vi "Halvorsen_ECD3_Fast.vi"(0 "tolerance":dbl=1e-13, 1 "Error Analysis":u16(ring)=4 items=["Max", "Max_Norm", "Norm", "Last Value", "Last Constant"], 3 "Шаг h, с":dbl=0.01, 4 "k":i32=4, 5 "Время, с":dbl=30.0, 7 "Hmax":dbl=1.0, 8 "b":dbl[](array[numeric])=[0.1, 0.1, 0.1], 10 "last_point_Thomas":dbl[](array[numeric])=[2.3727475682665875, 0.23609824454436878, 0.4447912442126299], 13 "Hmin":dbl=0.001, 15 "Points count":i32=2, 18 "n":i32[](array[numeric])=[2, 4, 6, 8, 10, 12, 14, 16, 18, 20, 22], 19 "Ext.Type":u16(ring) items=["FNode", "MathScript", "ECD8 Arrays", "ECD8 Fnode", "ECD8 FnodeDiv", "FNode Exp"]) -> (6 "Elapsed Time":dbl=0.0023101388233044418, 12 "Number of steps":i32=215, 14 "Error Estimation":dbl=7.276980385616179e-13, 17 "Rejected steps":i32=3)   [LabVIEW 2016]
uses:
  <vilib>/Analysis/_algsub.llb/Real Vector Norm.vi
  <vilib>/Analysis/5stat.llb/RMS (DBL).vi
  <vilib>/Analysis/NI_AALBase.lvlib
  <vilib>/Analysis/NI_AALPro.lvlib
panel:
  in  "Initial Conditions":dbl[](array[numeric])=[1.0, 0.0, 1.0]
  out "Last Value Reference":dbl[](array[numeric])=[2.372747587228327, 0.2360982570449824, 0.44479123342230803] format="%#_15f"
  out "Rejected Steps":i32[](graph)=[0, 0, 0, 0, 0, 0, 0, 0, 0, 0, 0, 0, 0, 0, 0, 0, 0, 0, 0, 0, 0, 0, 0, 0, 0, 0, 0, 0, 0, 0, 0, 0, 0, 0, 0, 0, 0, 0, 0, 0, 0, 0, 0, 0, 0, 0, 0, 0, 0, 0, 0, 0, 0, 0, 0, 0, 0, 0, 0, 0, 0, 0, 0, 0, 0, 0, 0, 0, 0, 0, 0, 0, 0, 0, 0, 0, 0, 0, 0, 0, 0, 0, 0, 0, 0, 0, 0, 0, 0, 0, 0, 0, 0, 0, 0, 0, 0, 0, 0, 0, 0, 0, 0, 0, 0, 0, 0, 0, 0, 0, 0, 0, 0, 0, 1, 0, 0, 0, 0, 0, 0, 0, 0, 0, 0, 0, 0, 0, 0, 0, 0, 0, 0, 0, 0, 0, 0, 0, 0, 0, 0, 0, 0, 0, 0, 0, 0, 0, 0, 0, 0, 0, 0, 0, 0, 0, 0, 0, 0, 0, 0, 0, 0, 0, 0, 0, 0, 0, 0, 0, 0, 0, 0, 0, 0, 0, 0, 0, 0, 0, 0, 0, 0, 0, 0, 0, 1, 0, 0, 0, 0, 1, 0, 0, 0, 0, 0, 0, 0, 0, 0, 0, 0, 0, 0, 0, 0, 0, 0, 0, 0, 0, 0, 0, 0, 0]
  out "Last Value":dbl[](array[numeric])=[2.3727475682670662, 0.2360982445444861, 0.44479124421209454] format="%#_15f"
  out "Step time variation":dbl[](graph)=[0.002410370462712308, 0.0022099071838965756]
  out "Real Error":dbl[][](graph)=[[0.0, 0.0, 0.0], [4.6629367034256575e-15, 1.908195823574488e-15, 1.7763568394002505e-15], [1.748490241482159e-12, 5.903055821931957e-13, 2.1094237467877974e-14], [5.741995767749586e-11, 1.6126516788617096e-11, 1.5851764345597985e-12], [2.8038460442303403e-10, 6.303146893316125e-11, 1.404787397518703e-11], [4.9621040609793e-10, 9.647355136976898e-11, 4.231348604832874e-11], [6.795632945255647e-10, 1.172824615203183e-10, 8.282352581545638e-11], [8.33989544091196e-10, 1.2820922101752785e-10, 1.3152390287984872e-10], [9.677894041715263e-10, 1.2962053652643135e-10, 1.8526247202999002e-10], [1.087936851718041e-09, 1.1890322060281733e-10, 2.4136426191034843e-10], [1.1999332638623628e-09, 8.893674685594988e-11, 2.966178413998932e-10], [1.2968486284847813e-09, 2.879207983141896e-11, 3.4188940567503323e-10], [1.3438086199357713e-09, -4.558087240980058e-11, 3.5787728336345026e-10], [1.3577134971853866e-09, -1.2493472922869842e-10, 3.432942818903939e-10], [1.354880652115753e-09, -2.1241652881087703e-10, 2.9695623737779897e-10], [1.3423706590742768e-09, -3.1278557521829953e-10, 2.0913804021915894e-10], [1.3237086982087476e-09, -4.3100079061275665e-10, 5.410383252524298e-11], [1.3041514534961607e-09, -5.177385187238315e-10, -1.521587300601368e-10], [1.2894871836977018e-09, -5.417550852371278e-10, -3.6701575112374485e-10], [1.2790746239943473e-09, -5.146085779728082e-10, -6.057510049117809e-10], [1.2707515040233375e-09, -4.3312020636676607e-10, -8.863207945353224e-10], [1.2613066147082463e-09, -2.8478619462646293e-10, -1.2270384708301663e-09], [1.2457230802453978e-09, -5.0502935167173746e-11, -1.6514722922522651e-09], [1.2178640318438738e-09, 2.7474467145793824e-10, -2.1226838065047104e-09], [1.173521724240345e-09, 6.642104644072333e-10, -2.548607991315066e-09], [1.1083001183465058e-09, 1.1039147373992364e-09, -2.922341035827003e-09], [1.017403494785185e-09, 1.5845043055406904e-09, -3.240587354014224e-09], [8.940710394256257e-10, 2.1000174932339633e-09, -3.5038705270551418e-09], [7.26753324187257e-10, 2.650429875572513e-09, -3.716026153455232e-09], [5.006035586063717e-10, 3.2262850169217927e-09, -3.8690446402256384e-09], [1.9380763660592493e-10, 3.816509774878796e-09, -3.955048732962041e-09], [-2.0528290178845054e-10, 4.372683548581335e-09, -3.95721366786006e-09], [-6.853815293084153e-10, 4.834492361993625e-09, -3.873784404362368e-09], [-1.231378554678031e-09, 5.183864892899237e-09, -3.718152896681204e-09], [-1.838136309828542e-09, 5.43066525082736e-09, -3.4995242259583392e-09], [-2.4965642886343176e-09, 5.583902229489013e-09, -3.2218598899902418e-09], [-3.20633031236639e-09, 5.655568013906986e-09, -2.8814779451380446e-09], [-3.95173493927814e-09, 5.653833845542522e-09, -2.475329274886917e-09], [-4.717421564492952e-09, 5.591174190300308e-09, -1.997236598327845e-09], [-5.481618714497927e-09, 5.484983578440961e-09, -1.4417773641639542e-09], [-6.222447002102172e-09, 5.3586233228486435e-09, -8.048868238574869e-10], [-6.927526552402696e-09, 5.2384971915842016e-09, -8.118239414045547e-11], [-7.589623596260253e-09, 5.152425153198692e-09, 7.313869510028326e-10], [-8.214809277262702e-09, 5.1254382960053135e-09, 1.639219426863292e-09], [-8.815759233726794e-09, 5.180855744413293e-09, 2.651973751710557e-09], [-9.412382873108527e-09, 5.342479347802964e-09, 3.7888571169375496e-09], [-1.0020086094186809e-08, 5.634394728559755e-09, 5.058699126259114e-09], [-1.0670280659041964e-08, 6.0878764251981465e-09, 6.5014074124292165e-09], [-1.1386144471714488e-08, 6.732222335159577e-09, 8.133392848108656e-09], [-1.2184061315423378e-08, 7.58216733842687e-09, 9.939812195547404e-09], [-1.3073527593832068e-08, 8.631241499301723e-09, 1.1878749317517645e-08], [-1.4058679997930312e-08, 9.855596339036765e-09, 1.3899611461809513e-08], [-1.5135776632035913e-08, 1.1216054751628235e-08, 1.5948250164932176e-08], [-1.6288862259017378e-08, 1.2655923420368254e-08, 1.7962675902261083e-08], [-1.748360478615041e-08, 1.4096415590358902e-08, 1.9864868083807607e-08], [-1.8675936797052373e-08, 1.5452399360071922e-08, 2.158286260822706e-08], [-1.9839095699580866e-08, 1.6667154767446846e-08, 2.3089951728394453e-08], [-2.095904472199095e-08, 1.7701697885286194e-08, 2.437547474976043e-08], [-2.201700777249016e-08, 1.8510371013746862e-08, 2.5409759407679644e-08], [-2.300580370651062e-08, 1.904587509926614e-08, 2.615640637415595e-08], [-2.3907172241877106e-08, 1.922074766014248e-08, 2.6519400453395292e-08], [-2.4576130464026846e-08, 1.8954913194590972e-08, 2.634338214235754e-08], [-2.499571194469752e-08, 1.8347311225852536e-08, 2.5702095118873558e-08], [-2.5227674615990736e-08, 1.746203803776325e-08, 2.4635880668810728e-08], [-2.5297896444342882e-08, 1.634465718325373e-08, 2.3138052585025548e-08], [-2.521778097452909e-08, 1.4991229591032607e-08, 2.1085527102115975e-08], [-2.4980785218176038e-08, 1.342938471537991e-08, 1.8295216452912655e-08], [-2.4565228740058842e-08, 1.1723129134111332e-08, 1.4375302725966321e-08], [-2.410824262444322e-08, 1.0450478704626676e-08, 1.0731142197073495e-08], [-2.3612022115315767e-08, 9.507560960742012e-09, 7.059913542661889e-09], [-2.3075088118051923e-08, 8.896805070435221e-09, 3.3140565847133985e-09], [-2.2496197252253047e-08, 8.635524295641517e-09, -4.3445602670999506e-10], [-2.1872917907450606e-08, 8.713377575020331e-09, -4.052451263447665e-09], [-2.1195635607762497e-08, 9.07830965957146e-09, -7.431223636444884e-09], [-2.0436776437815496e-08, 9.656937471902438e-09, -1.0555558649372188e-08], [-1.9566793074687894e-08, 1.0352647628053546e-08, -1.3387417174826055e-08], [-1.8554563219197462e-08, 1.1040079961333049e-08, -1.5889236149035924e-08], [-1.7441594835077012e-08, 1.1531731125558053e-08, -1.78981196530259e-08], [-1.6287802995229583e-08, 1.1705465041700336e-08, -1.9404356788044197e-08], [-1.509272262723016e-08, 1.1515045805765567e-08, -2.0542217260555162e-08], [-1.3864163594945467e-08, 1.090078249887938e-08, -2.1392820404031454e-08], [-1.2602452192922442e-08, 9.73826619343754e-09, -2.2016690914838932e-08], [-1.1385494103066662e-08, 7.872688279064732e-09, -2.2424265333498283e-08], [-1.0442427367252094e-08, 5.584611884046353e-09, -2.260593667813282e-08], [-9.809990819675818e-09, 3.0103626258437544e-09, -2.263313902961528e-08], [-9.492732377935909e-09, 1.3581935576212345e-10, -2.2549517031400512e-08], [-9.520266575080427e-09, -3.0369680104058716e-09, -2.23705429736043e-08], [-9.93233650881109e-09, -6.5029741591615675e-09, -2.2091959317460663e-08], [-1.0751474155412666e-08, -1.015298156659128e-08, -2.1694960022911047e-08], [-1.1850443293326407e-08, -1.3503982820850524e-08, -2.118631035018248e-08], [-1.3036269175259463e-08, -1.6347810216643666e-08, -2.0578504067447767e-08], [-1.4216547938872282e-08, -1.88094659847593e-08, -1.9848522991861017e-08], [-1.5334836067637525e-08, -2.0992553473320186e-08, -1.895512730110127e-08], [-1.6322717844019508e-08, -2.2945967792509236e-08, -1.784551412198354e-08], [-1.709702290852988e-08, -2.4732368153479456e-08, -1.6410588554727212e-08], [-1.7423020359785824e-08, -2.6162587651867852e-08, -1.4742066789530384e-08], [-1.7226773785239402e-08, -2.7146626280227792e-08, -1.308614105965944e-08], [-1.654973891263012e-08, -2.7845280747840206e-08, -1.1417249257128503e-08], [-1.5346170556540528e-08, -2.8334817159247905e-08, -9.72335079119091e-09], [-1.3519495745129007e-08, -2.8647375138746156e-08, -8.042690180509737e-09], [-1.0812458040021511e-08, -2.8804419294203853e-08, -6.415972420015237e-09], [-7.400701385051889e-09, -2.881414262745352e-08, -5.131944424974222e-09], [-3.744289767126929e-09, -2.872946991416825e-08, -4.357797678267161e-09], [1.2021139639273315e-10, -2.8598414747449397e-08, -4.0738965534359295e-09], [4.026620814556736e-09, -2.8456553113898053e-08, -4.2714742853888765e-09], [7.845780025661497e-09, -2.8329004475580177e-08, -4.9125035150865415e-09], [1.1536529953559693e-08, -2.822989308981505e-08, -5.955672621738017e-09], [1.5163314159849506e-08, -2.8164639065408892e-08, -7.3979775638832734e-09], [1.8703919746343445e-08, -2.8133652296702394e-08, -9.232929976121795e-09], [2.1937712535446963e-08, -2.8125184403648973e-08, -1.1337834227020949e-08], [2.4605244508535407e-08, -2.8111044603207347e-08, -1.3457895686741495e-08], [2.6779117145991904e-08, -2.8057470569109455e-08, -1.549388284338704e-08], [2.8548334363165395e-08, -2.7926878587436477e-08, -1.740889099544063e-08], [2.9952631930285634e-08, -2.7670322033657158e-08, -1.9165770526186066e-08], [3.10083656529514e-08, -2.7202047947483265e-08, -2.0741275363889145e-08], [3.150672345242356e-08, -2.6550981635509174e-08, -2.176558044908461e-08], [3.157240247020354e-08, -2.567057189040156e-08, -2.23203409088768e-08], [3.125887815258466e-08, -2.461792436569965e-08, -2.23818592548497e-08], [3.06181016096474e-08, -2.3368021961900354e-08, -2.1991309218094557e-08], [2.963904321973132e-08, -2.187334513514827e-08, -2.1113139236916822e-08], [2.8083123826405654e-08, -1.9865920242168045e-08, -1.9427071062949608e-08], [2.6548995668562725e-08, -1.8074725938177494e-08, -1.757328371709832e-08], [2.5073919607265793e-08, -1.6481428222192562e-08, -1.5662415364658955e-08], [2.358768635968289e-08, -1.499975343932647e-08, -1.3634921636196395e-08], [2.207516958119271e-08, -1.3628246198216232e-08, -1.1488191287156724e-08], [2.0525785848768408e-08, -1.2386289882648782e-08, -9.227639097275642e-09], [1.8927614475749976e-08, -1.130792448567064e-08, -6.867263646626043e-09], [1.7284886133506205e-08, -1.0447979148509035e-08, -4.464005609605692e-09], [1.560497603358968e-08, -9.858254157446567e-09, -2.10127115707337e-09], [1.3894552397530902e-08, -9.569756154181874e-09, 1.252487003000624e-10], [1.2105056623745725e-08, -9.584839255616373e-09, 2.179602276441983e-09], [1.0165710717657817e-08, -9.902505426762076e-09, 4.0250411892372995e-09], [7.971655335836658e-09, -1.052305963200606e-08, 5.6118745206390486e-09], [5.2726414345727335e-09, -1.1477731908296745e-08, 6.8749126391765e-09], [2.2244107389379764e-09, -1.2636918358954752e-08, 7.543660363040772e-09], [-5.508475620086273e-10, -1.3690120259646221e-08, 7.553732750409381e-09], [-3.204670639966878e-09, -1.4613361243309697e-08, 7.063207796420556e-09], [-5.782402057175062e-09, -1.537909566362572e-08, 6.138056729554364e-09], [-8.281175301050325e-09, -1.5950971765654742e-08, 4.820918331205348e-09], [-1.0683739448680285e-08, -1.628644630269349e-08, 3.151491512198845e-09], [-1.2940178373277433e-08, -1.6335645280918243e-08, 1.2021827977548583e-09], [-1.496146473378701e-08, -1.6066944774628666e-08, -8.757892189237282e-10], [-1.671627902766204e-08, -1.5485193349817905e-08, -2.9468196771631483e-09], [-1.8229253107016063e-08, -1.46013214852303e-08, -4.943017994918364e-09], [-1.9531423700591688e-08, -1.3415870525612661e-08, -6.827112208895869e-09], [-2.0649502330272185e-08, -1.1907022035018144e-08, -8.579156052235248e-09], [-2.1581062936704143e-08, -1.0060293487157423e-08, -1.0151148810422228e-08], [-2.2294190937799385e-08, -7.91925458543119e-09, -1.1460428606113737e-08], [-2.2739666372117995e-08, -5.690775406463899e-09, -1.2404139049237983e-08], [-2.291839540369267e-08, -3.5313562074534843e-09, -1.2990837294779567e-08], [-2.2847095992872823e-08, -1.4838082984525158e-09, -1.3282665189962017e-08], [-2.2531094989730605e-08, 4.2930836663401806e-10, -1.3336230342275712e-08], [-2.1967723418114815e-08, 2.1931216287462973e-09, -1.3203070192702171e-08], [-2.115066055630166e-08, 3.797658576498719e-09, -1.29329857934124e-08], [-2.0055410665520412e-08, 5.2549363194209775e-09, -1.2571880869671759e-08], [-1.8631638676325224e-08, 6.5799804493948955e-09, -1.2164275808856928e-08], [-1.684925465816889e-08, 7.757980882705517e-09, -1.1767410157403901e-08], [-1.510724767506133e-08, 8.635000464662923e-09, -1.1476723571490766e-08], [-1.3486575412002821e-08, 9.27923643478934e-09, -1.1297882629435207e-08], [-1.1949769840313706e-08, 9.76447722678131e-09, -1.1214004835835567e-08], [-1.0471833178371526e-08, 1.0129247385304296e-08, -1.1210403272343683e-08], [-9.035652670519312e-09, 1.0392698590599991e-08, -1.12725535572622e-08], [-7.606012042415955e-09, 1.0562990815365936e-08, -1.138181104920477e-08], [-6.1661398209622575e-09, 1.0632352664963207e-08, -1.1499670549142138e-08], [-5.000995839665734e-09, 1.059520149393478e-08, -1.1595077786807906e-08], [-4.124830588203565e-09, 1.0484104251418103e-08, -1.1664643473352498e-08], [-3.4429135098434926e-09, 1.0319303633821164e-08, -1.1693638946042029e-08], [-2.9191853379018085e-09, 1.0112433779241314e-08, -1.1664394783394982e-08], [-2.5477085996428173e-09, 9.875305018169911e-09, -1.1552974577000441e-08], [-2.3485392519617676e-09, 9.631408559584997e-09, -1.13574980531439e-08], [-2.3340464838650377e-09, 9.427337355205623e-09, -1.1200794958199367e-08], [-2.4710480467371454e-09, 9.282342006144972e-09, -1.1102374131155557e-08], [-2.7482891171159984e-09, 9.21065779202479e-09, -1.1054524406972632e-08], [-3.1753725482364104e-09, 9.233186215595879e-09, -1.1063286287082974e-08], [-3.7314135670207804e-09, 9.368881670468454e-09, -1.1172207159404479e-08], [-4.366740968819727e-09, 9.61946433619687e-09, -1.1391810161853755e-08], [-5.087907484213616e-09, 9.990131388804002e-09, -1.1696436708064084e-08], [-5.919705836632261e-09, 1.0494234370383992e-08, -1.2080000111325262e-08], [-6.895876536461287e-09, 1.114836001292474e-08, -1.2549684846874243e-08], [-8.039838128581778e-09, 1.1961454937647886e-08, -1.3113800267916531e-08], [-9.281615476197658e-09, 1.2928445425330892e-08, -1.3738790549666646e-08], [-1.0613240619683495e-08, 1.4041897422600869e-08, -1.4405312942500359e-08], [-1.2062517318334187e-08, 1.5293519783909915e-08, -1.5113948315104153e-08], [-1.3654044450639446e-08, 1.6671918512400907e-08, -1.586661513286458e-08], [-1.540142857692217e-08, 1.815647010516841e-08, -1.6659772672511508e-08], [-1.7307913102726502e-08, 1.9710232557201834e-08, -1.7482377323574383e-08], [-1.9398786799129653e-08, 2.1244638048756315e-08, -1.8325109429895292e-08], [-2.1078749412595243e-08, 2.2736189819738684e-08, -1.8935185863711013e-08], [-2.2668807719838924e-08, 2.4123604891457262e-08, -1.9420713481821394e-08], [-2.4020089695042657e-08, 2.5324322194819615e-08, -1.9716681176618067e-08], [-2.5135232561979137e-08, 2.6319593171564293e-08, -1.9809717421992445e-08], [-2.5989247864899312e-08, 2.7087934340030984e-08, -1.9657945937723298e-08], [-2.6486870030595355e-08, 2.757895978255931e-08, -1.920834447055597e-08], [-2.6560774468720183e-08, 2.7767683707935475e-08, -1.843999197781443e-08], [-2.6242586992353267e-08, 2.7693558557473352e-08, -1.747519196015901e-08], [-2.5562321370742325e-08, 2.7395669732754868e-08, -1.629851720252873e-08], [-2.4489656524906422e-08, 2.6884801718196627e-08, -1.487597245386496e-08], [-2.287958134061796e-08, 2.612616301078674e-08, -1.3066682180706835e-08], [-2.1033863983888068e-08, 2.5302803186022516e-08, -1.1308157743528113e-08], [-1.907247604293616e-08, 2.4487197380906878e-08, -9.678039925020698e-09], [-1.695272411339488e-08, 2.3678520477687925e-08, -8.120355055041273e-09], [-1.465069976447353e-08, 2.2887666206727886e-08, -6.6375835938714545e-09], [-1.213586564574598e-08, 2.2127724430553997e-08, -5.252195123262027e-09], [-9.336648787439117e-09, 2.1409510386760644e-08, -3.994404917939676e-09], [-6.3154490526073914e-09, 2.076679272988713e-08, -2.986116798275873e-09], [-3.385290270330188e-09, 2.0218216323364402e-08, -2.3670400639552724e-09], [-5.577565076464452e-10, 1.9725117178515106e-08, -2.1045847287126662e-09], [2.193686121643168e-09, 1.924452749935135e-08, -2.1692057039501833e-09], [4.87828355488773e-09, 1.8733983822571965e-08, -2.5436720785254607e-09], [7.484302066984583e-09, 1.815157417428548e-08, -3.2121523774186755e-09], [1.000124294492366e-08, 1.745529717989136e-08, -4.159933161829166e-09], [1.2412752603552235e-08, 1.660475872078404e-08, -5.3737923416674604e-09], [1.4685198390651522e-08, 1.5566174099701513e-08, -6.835208649080826e-09], [1.6765431709586665e-08, 1.432168855730609e-08, -8.511302607150384e-09], [1.8600188500528247e-08, 1.2874491334136096e-08, -1.0361099367361959e-08], [1.896126056166736e-08, 1.2500496304745923e-08, -1.0789786508702548e-08]]
  out "Step Variation":dbl[](graph)=[0.01, 0.04231663774973586, 0.09882701022120709, 0.13702631818436026, 0.13418628920067735, 0.1289180839074337, 0.1252240367028919, 0.12419212185082452, 0.12624692311830657, 0.13213044935422963, 0.13956309064513636, 0.1348085010848226, 0.1297832850982968, 0.13049049802490806, 0.13704713448397493, 0.15030074724249978, 0.15357889771541217, 0.14733026447078357, 0.14772106506695848, 0.15332079825567016, 0.16254246102292572, 0.1750582839592434, 0.18223488210606506, 0.17813475088242853, 0.17389626519253076, 0.16989005060861676, 0.16690026804232672, 0.16638316205167397, 0.16633707651581764, 0.16754513116297085, 0.164939046918228, 0.15701158402544957, 0.14842285398452099, 0.14253284305720457, 0.1383876843022662, 0.13709877336899942, 0.13636793480065174, 0.13641752672563756, 0.13637328082024333, 0.1357942096442934, 0.13507206452361467, 0.133825908652664, 0.13300544249367913, 0.13299041996363817, 0.13459367675944586, 0.13642557287187423, 0.1410042620781306, 0.1458351394905747, 0.1491327412641486, 0.15018524983015258, 0.14947739826937703, 0.14753343228368618, 0.14446934558940833, 0.1397694868513425, 0.13371408018116143, 0.12874166190634762, 0.1262829272810691, 0.1260693836172068, 0.13030173047424473, 0.1402302949057107, 0.13608220608483054, 0.125319993314077, 0.1223112084340788, 0.12295983814436025, 0.1308931956608282, 0.14433169129385864, 0.16683503737746483, 0.14894268611000228, 0.144970570787907, 0.14571231992017994, 0.14722651475761392, 0.14751515749550753, 0.14685563928247872, 0.14797168432794236, 0.15013851254586333, 0.15336091710513616, 0.14958371886309682, 0.14141023251428148, 0.1379723629604659, 0.13872865137066323, 0.14624672147125803, 0.156226754537656, 0.14961575242204248, 0.14327424032595104, 0.14222740560544353, 0.1442468657130614, 0.1488324122933823, 0.15308948166527744, 0.14607894890625275, 0.13379649481789382, 0.12631331915466537, 0.12395540587942071, 0.1256636008657248, 0.13444983300717817, 0.13463120061364167, 0.12257819136419408, 0.11827314060966711, 0.1198537420976382, 0.12509327870669998, 0.1374987373787398, 0.1408574485053432, 0.1345453051049277, 0.13176323806068638, 0.1282324479505426, 0.1243615412926346, 0.12175570779816948, 0.12287134192086151, 0.12569930908832688, 0.12489691856802153, 0.11735988867446111, 0.11175307838779279, 0.10991723743294135, 0.11188624693760468, 0.12082859922232835, 0.12752646131111778, 0.11291375799237935, 0.1083284264750177, 0.10947454126195574, 0.11643704593555175, 0.14322473074635453, 0.127688171829751, 0.11799001621854179, 0.11752788185142204, 0.12075360377696083, 0.12672591146017442, 0.13510783353564593, 0.1440120117597863, 0.15208997474192815, 0.15806433568582562, 0.1654208914649322, 0.17513428488561125, 0.18882405728501997, 0.21461881380420067, 0.22536098860505824, 0.20008811571766166, 0.18755083723488516, 0.18125499871147385, 0.17814515452442156, 0.17733611366432253, 0.176473065520423, 0.1714614059607094, 0.16460725741916127, 0.15970693650684042, 0.15783521391091027, 0.16008672783113562, 0.16489712919260913, 0.16912628010715194, 0.16521838232164293, 0.15777213835157544, 0.15244006476779107, 0.14920303370844928, 0.14767753694752128, 0.14754247301942178, 0.15025625219779754, 0.15657218181574595, 0.1640172761335006, 0.15076245987883585, 0.1378711380873641, 0.13074020097776679, 0.12784843357949463, 0.12855003624568265, 0.1344886960864465, 0.14555696493482181, 0.13912147988980422, 0.12890528196814094, 0.1259702229430159, 0.12797979689064898, 0.13392852143189918, 0.14024180615245135, 0.1351702333997724, 0.13105943367932868, 0.1314981244158217, 0.13553459651205915, 0.13510351871152604, 0.12854624823253336, 0.12556237142132873, 0.12671509752070717, 0.1314847094987767, 0.13754868665000103, 0.1347077061889213, 0.13079127679206076, 0.1295564048797411, 0.13065883225941163, 0.13364747171342992, 0.1390205444412019, 0.1517501574429627, 0.14186091852936328, 0.12413945633187237, 0.11704297005526362, 0.1151072107210323, 0.11969748924349469, 0.1441194468341694, 0.12493054200333974, 0.11315506510474135, 0.11213026429606998, 0.11784593825441098, 0.13758823644464394, 0.12693235381129037, 0.11792110060883987, 0.11787024531202452, 0.12200671651440423, 0.12970897490656463, 0.14287890404272854, 0.15371989865300575, 0.1489712621230145, 0.1455729192658614, 0.1448726331446601, 0.14576928240911993, 0.14718930022560528, 0.14937156790311482, 0.1522729807219658, 0.15512988119548488, 0.1566791798916945, 0.15650511870511, 0.03445178495197254, 0.0]
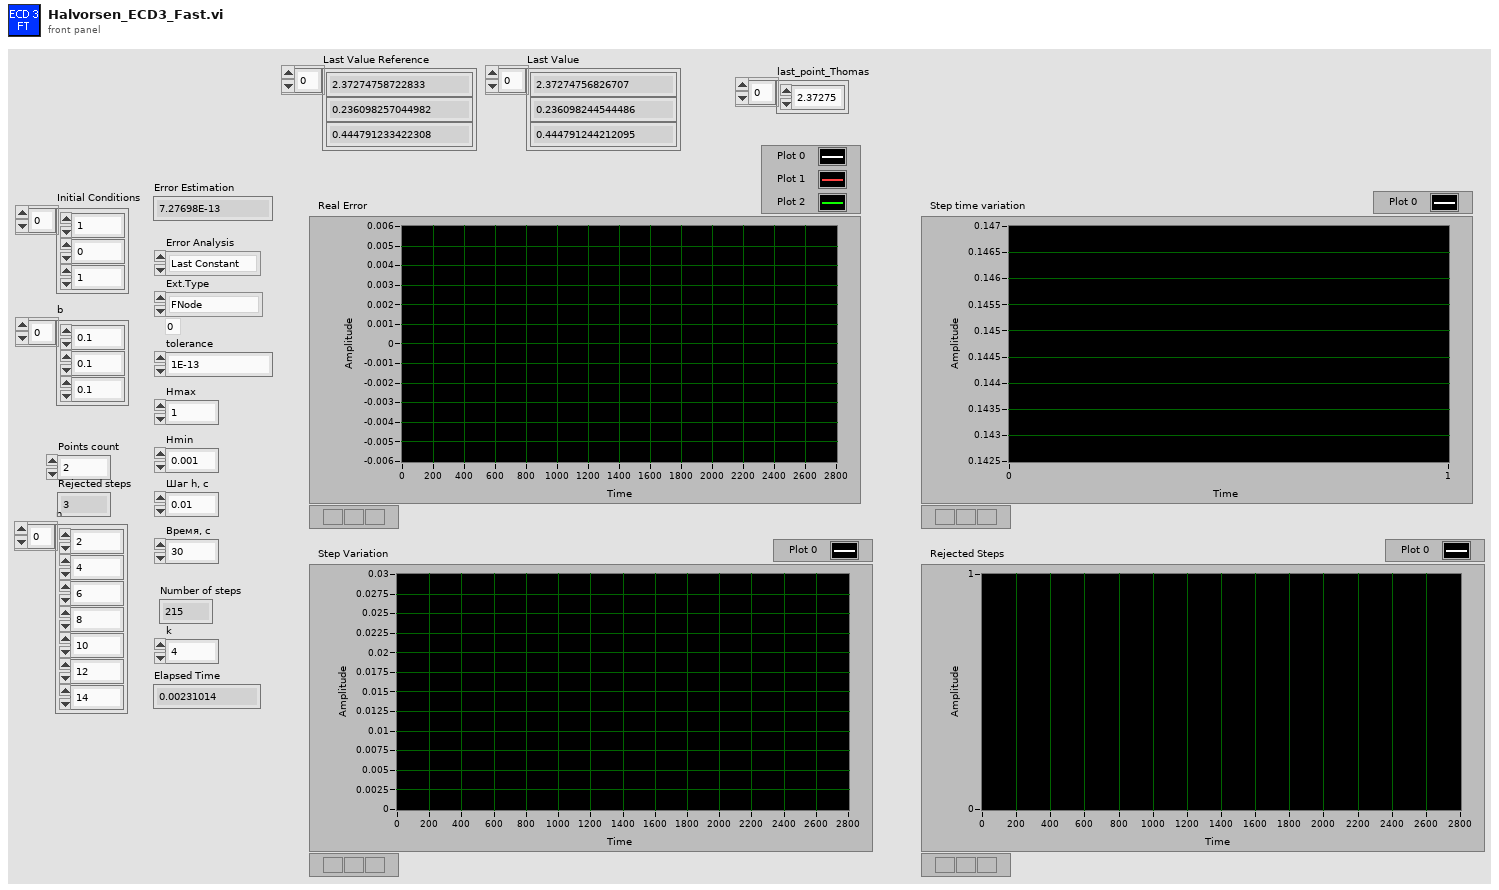
[diagram p1: front panel]
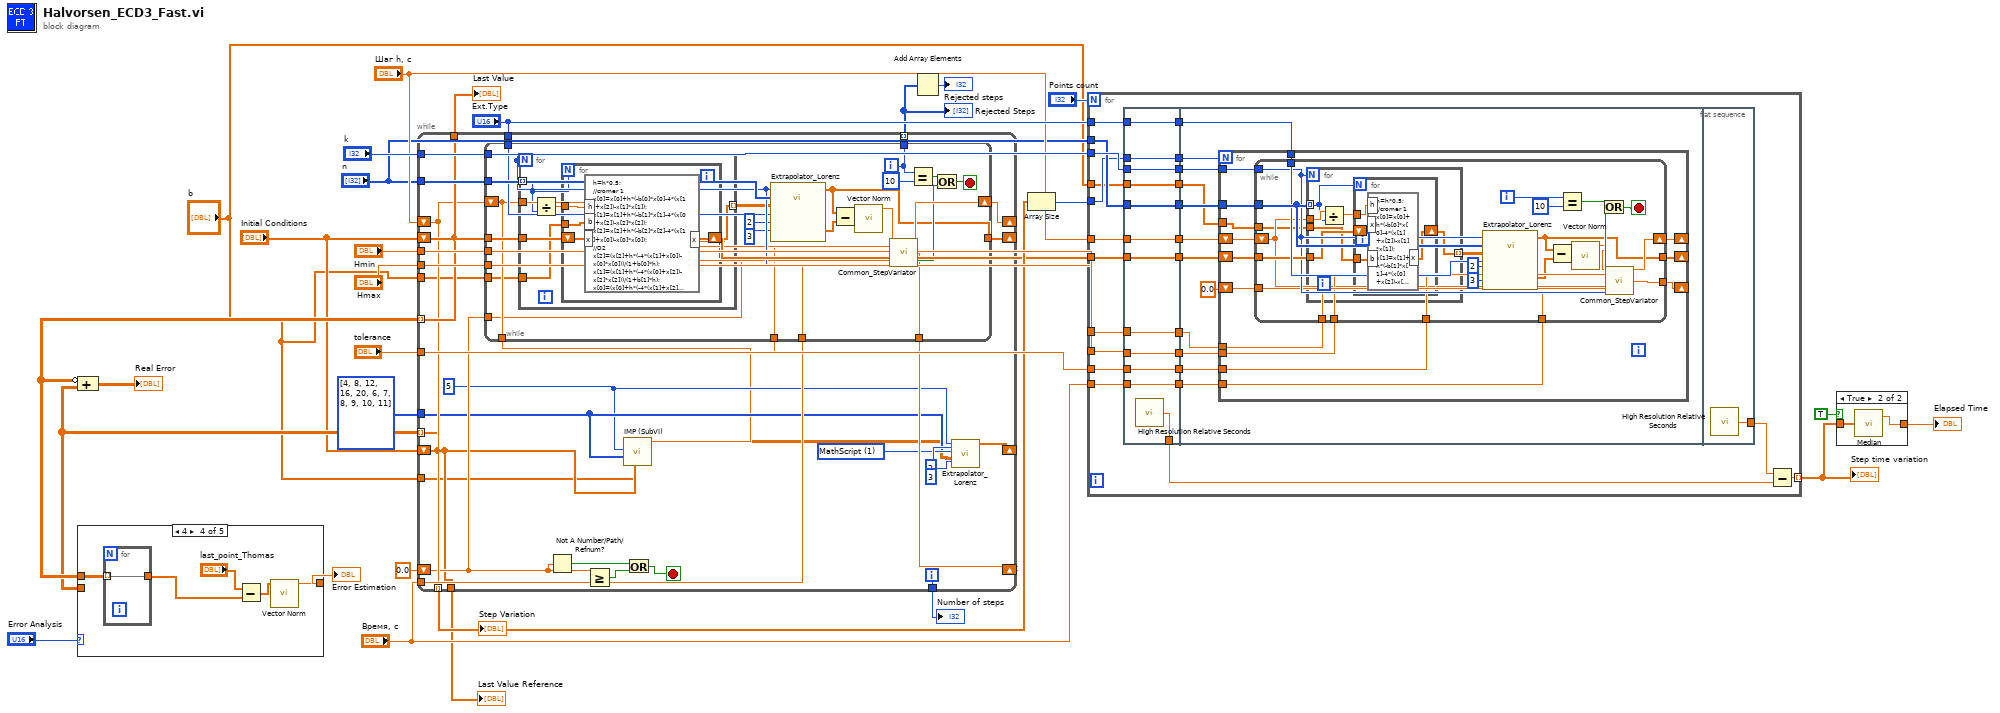
[diagram p0: block diagram]
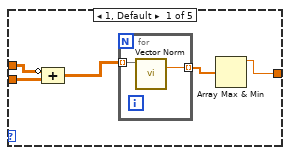
[diagram p2: hidden frame]
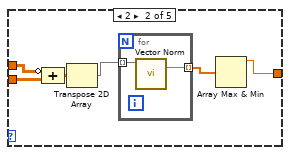
[diagram p3: hidden frame]
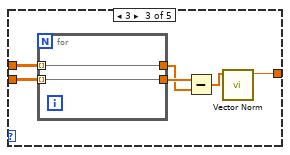
[diagram p4: hidden frame]
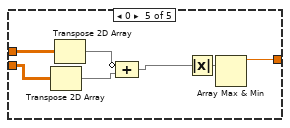
[diagram p5: hidden frame]
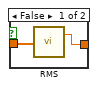
[diagram p6: hidden frame]
diagram:
  n1 = while {
    shift-right: [w50] -> _
    shift-left: "Initial Conditions" -> [w43]
    tunnel: "n" -> [w57]
    tunnel: "k" -> [w55]
    tunnel: "Ext.Type" -> [w46]
    shift-right: [w54] -> _
    shift-left: "Шаг h, с" -> [w37]
    shift-right: [w45] -> _
    shift-left: 0.0 -> [w36]
    tunnel: [w37] -> w13 mode=indexing
    tunnel: "Время, с" -> [w44]
    tunnel: [w56] -> w23
    tunnel: "tolerance" -> [w51]
    tunnel: "Hmin" -> [w53]
    tunnel: "Hmax" -> [w52]
    tunnel: [w43] -> w6 mode=indexing
    shift-right: [w49] -> _
    shift-left: "Initial Conditions" -> [w32]
    tunnel: i32[] [4, 8, 12, 16, 20, 6, 7, 8, 9, 10, 11] ("n 2") -> [w34]
    tunnel: [w32] -> w5 mode=indexing
    tunnel: [w43] -> w11
    tunnel: [w42] -> w10 mode=indexing
    tunnel: [w32] -> w4
    tunnel: "b" -> [w30]
    tunnel: "b" -> [w35]
    i -> [w56]
    stop <- w38 stop-if-true
    w41 = u16 1 items=["FNode", "MathScript", "ECD8 Arrays", "ECD8 Fnode", "ECD8 FnodeDiv"] ("Ext.Type")
    w33 = 5
    n2 = while {
      tunnel: w57 -> [w82]
      tunnel: w55 -> [w81]
      tunnel: w53 -> [w79]
      tunnel: w52 -> [w78]
      tunnel: w51 -> [w77]
      tunnel: [w60] -> w50
      tunnel: w46 -> [w73]
      tunnel: [w64] -> w45
      tunnel: w44 -> [w72]
      tunnel: w43 -> [w71]
      shift-right: [w80] -> w54
      shift-left: w37 -> [w66]
      tunnel: [w66] -> w31
      tunnel: [w65] -> w42
      tunnel: w36 -> [w63]
      tunnel: w35 -> [w62]
      i -> [w65]
      stop <- w68 stop-if-true
      n3 = for {
        N: w81 -> [_]
        tunnel: w82 -> [w85] mode=indexing
        tunnel: w66 -> [w86]
        tunnel: w71 -> [w88]
        tunnel: [w87] -> w74 mode=indexing
        tunnel: w62 -> [w83]
        n4 = Divide(x=w86, y=w85) -> (x/y=w84:dbl)
        n5 = for {
          N: w85 -> [_]
          shift-right: [w91] -> w87
          shift-left: w88 -> [w92]
          tunnel: w84 -> [w90]
          tunnel: w83 -> [w89]
          n6 = formula code="h=h*0.5;\n//cromer 1\nx[0]=x[0]+h*(-b[0]*x[0]-4*(x[1]+x[2])-x[1]*x[1]);\nx[1]=x[1]+h*(-b[1]*x[1]-4*(x[0]+x[2])-x[2]*x[2]);\nx[2]=x[2]+h*(-b[2]*x[2]-4*(x[1]+x[0])-x[0]*x[0]);\n//D2\nx[2]=(x[2]+h*(-4*(x[1]+x[0])-x[0]*x[0]))/(1+b[0]*h);\nx[1]=(x[1]+h*(-4*(x[0]+x[2])-x[2]*x[2]))/(1+b[1]*h);\nx[0]=(x[0]+h*(-4*(x[1]+x[2])-x[1]*x[1]))/(1+b[2]*h);"("x"=w92, "h"=w90, "b"=w89) -> ("x"=w91:dbl[])
        }
      }
      n7 = call "Extrapolator_Lorenz.vi"("Порядок экстраполятора"=2 ("input variable"), "Dimension"=3 ("input variable"), "Ext.Type"=w73, "Х - нач. условия"=w74, "n"=w82, "k"=w81) -> ("TPrev"=w59:dbl[], "Tout"=w60:dbl[])  [unwired: 4 in]
      n8 = Subtract(x=w60, y=w59) -> (x-y=w61:dbl[])
      n9 = call-poly <vilib>:"Vector Norm.vi"("Input Vector"=w61) -> ("norm"=w58:dbl)  [unwired: 9 in, 1 out]
      n10 = call "Common_StepVariator.vi"("err"=w58, "tolerance"=w77, "Hmax"=w78, "Шаг h, с"=w66, "Current time"=w63, "k"=w81, "Hmin"=w79, "tmax"=w72) -> ("Hnew"=w80:dbl, "New time"=w64:dbl, "stop"=w67:bool)  [unwired: 4 in, 1 out]
      n11 = Equal?(x=w65, y=10) -> (x = y?=w70:bool)
      n12 = Or(x=w70, y=w67) -> (x .or. y?=w68:bool)
    }
    n13 = Not A Number/Path/Refnum?(number/path/refnum=w36) -> (NaN/Path/Refnum?=w40:bool)
    n14 = Greater Or Equal?(x=w36, y=w44) -> (x >= y?=w39:bool)
    n15 = call "IMP (SubVI).vi"("Initial Conditions in"=w32, "b"=w30, "n in"=w34, "Numeric"=w33, "Шаг h, с"=w31) -> ("Initial Conditions out"=w29:dbl[][])  [unwired: 6 in]
    n16 = Or(x=w40, y=w39) -> (x .or. y?=w38:bool)
    n17 = call "Extrapolator_Lorenz.vi"("Порядок экстраполятора"=2, "Dimension"=3, "Ext.Type"=w41, "Х - нач. условия"=w29, "n"=w34, "k"=w33) -> ("Tout"=w49:dbl[])  [unwired: 4 in, 1 out]
  }
  "Step Variation" <- w13
  "Number of steps" <- w23
  "Last Value" <- w11
  "Rejected Steps" <- w10
  "Last Value Reference" <- w4
  n18 = Compound Arithmetic op=ADD(invert w6, w5) -> (→"Real Error":dbl[][])
  n19 = case shown="4" "Error Analysis" {
    tunnel: w5 -> [w94 w102 w111 _ w122]
    tunnel: [w96 w104 w113 w120 w127] -> w8
    tunnel: w6 -> [w95 w103 w112 w119 w123]
    frame 1, Default {
      n20 = Compound Arithmetic op=ADD(invert w95, w94) -> (w93:dbl[][])
      n21 = for {
        tunnel: [w99] -> w97 mode=indexing
        tunnel: w93 -> [w98] mode=indexing
        n22 = call-poly <vilib>:"Vector Norm.vi"("Input Vector"=w98) -> ("norm"=w99:dbl)  [unwired: 9 in, 1 out]
      }
      n23 = Array Max & Min(array=w97) -> (max value=w96:dbl)  [unwired: 3 out]
    }
    frame 2 {
      n24 = Compound Arithmetic op=ADD(invert w103, w102) -> (w101:dbl[][])
      n25 = Transpose 2D Array(2D array=w101) -> (transposed array=w100:dbl[][])
      n26 = for {
        tunnel: [w107] -> w105 mode=indexing
        tunnel: w100 -> [w106] mode=indexing
        n27 = call-poly <vilib>:"Vector Norm.vi"("Input Vector"=w106) -> ("norm"=w107:dbl)  [unwired: 9 in, 1 out]
      }
      n28 = Array Max & Min(array=w105) -> (max value=w104:dbl)  [unwired: 3 out]
    }
    frame 3 {
      n29 = for {
        tunnel: w112 -> [w115] mode=indexing
        tunnel: [w115] -> w109
        tunnel: w111 -> [w114] mode=indexing
        tunnel: [w114] -> w110
      }
      n30 = Subtract(x=w110, y=w109) -> (x-y=w108:dbl[])
      n31 = call-poly <vilib>:"Vector Norm.vi"("Input Vector"=w108) -> ("norm"=w113:dbl)  [unwired: 9 in, 1 out]
    }
    frame 4 {
      n32 = for {
        tunnel: w119 -> [w121] mode=indexing
        tunnel: [w121] -> w118
      }
      n33 = Subtract(x="last_point_Thomas", y=w118) -> (x-y=w117:dbl[])
      n34 = call-poly <vilib>:"Vector Norm.vi"("Input Vector"=w117) -> ("norm"=w120:dbl)  [unwired: 9 in, 1 out]
    }
    frame 0 {
      n35 = Transpose 2D Array(2D array=w122) -> (transposed array=w125:dbl[][])
      n36 = Transpose 2D Array(2D array=w123) -> (transposed array=w126:dbl[][])
      n37 = Compound Arithmetic op=ADD(invert w126, w125) -> (w124:dbl[][])
      n38 = Absolute Value(x=w124) -> (abs(x)=w128:dbl[][])
      n39 = Array Max & Min(array=w128) -> (max value=w127:dbl)  [unwired: 3 out]
    }
  }
  "Error Estimation" <- w8
  n40 = Add Array Elements(numeric array=w10) -> (sum=→"Rejected steps":i32)
  n41 = Array Size(array=w13) -> (size(s)=w22:i32)
  n42 = for {
    N: "Points count" -> [_]
    tunnel: "k" -> [w153]
    tunnel: "n" -> [w152]
    tunnel: "Ext.Type" -> [w132]
    tunnel: "Initial Conditions" -> [w151]
    tunnel: w22 -> [w150]
    tunnel: [w143] -> w20 mode=indexing
    tunnel: "Шаг h, с" -> [w134]
    tunnel: "Hmin" -> [w142]
    tunnel: "Hmax" -> [w139]
    tunnel: "tolerance" -> [w138]
    tunnel: "Время, с" -> [w136]
    tunnel: "b" -> [w129]
    n43 = flat-sequence {
      tunnel: w150 -> [w162]
      tunnel: w151 -> [w163]
      tunnel: w152 -> [w164]
      tunnel: w153 -> [w165]
      tunnel: [w165] -> w149
      tunnel: [w164] -> w148
      tunnel: [w163] -> w147
      tunnel: [w162] -> w146
      tunnel: [w161] -> w144
      tunnel: w142 -> [w160]
      tunnel: [w160] -> w141
      tunnel: w139 -> [w159]
      tunnel: [w159] -> w140
      tunnel: w138 -> [w158]
      tunnel: [w158] -> w137
      tunnel: w136 -> [w157]
      tunnel: [w157] -> w135
      tunnel: w134 -> [w156]
      tunnel: [w156] -> w133
      tunnel: w132 -> [w155]
      tunnel: [w155] -> w131
      tunnel: [w154] -> w130
      tunnel: w129 -> [w154]
      tunnel: w149 -> [w177]
      tunnel: w148 -> [w176]
      tunnel: w147 -> [w175]
      tunnel: w146 -> [w174]
      tunnel: w141 -> [w172]
      tunnel: w140 -> [w171]
      tunnel: w137 -> [w170]
      tunnel: w135 -> [w169]
      tunnel: w133 -> [w168]
      tunnel: w131 -> [w167]
      tunnel: w130 -> [w166]
      tunnel: [w227] -> w145
      frame #0 {
        n44 = call <vilib>:"High Resolution Relative Seconds.vi"() -> ("relative seconds"=w161:dbl)
      }
      frame #1 {
        n45 = for {
          N: w174 -> [_]
          shift-right: [w188] -> _
          shift-left: w175 -> [w179]
          tunnel: w176 -> [w191]
          tunnel: w177 -> [w187]
          tunnel: w167 -> [w190]
          shift-right: [w189] -> _
          shift-left: w168 -> [w182]
          tunnel: w172 -> [w186]
          tunnel: w171 -> [w185]
          tunnel: w170 -> [w184]
          shift-right: [w181] -> _
          shift-left: 0.0 -> [w180]
          tunnel: w169 -> [w183]
          tunnel: w166 -> [w178]
          n46 = while {
            tunnel: w191 -> [w216]
            tunnel: w190 -> [w215]
            tunnel: w179 -> [w214]
            tunnel: [w194] -> w188
            tunnel: w187 -> [w209]
            tunnel: w186 -> [w208]
            tunnel: w185 -> [w207]
            tunnel: w184 -> [w206]
            tunnel: w180 -> [w205]
            tunnel: w183 -> [w204]
            shift-right: [w210] -> w189
            shift-left: w182 -> [w197]
            tunnel: [w198] -> w181
            tunnel: w178 -> [w196]
            i -> [w200]
            stop <- w201 stop-if-true
            n47 = for {
              N: w209 -> [_]
              tunnel: w216 -> [w219] mode=indexing
              tunnel: w197 -> [w220]
              tunnel: w214 -> [w222]
              tunnel: [w221] -> w211 mode=indexing
              tunnel: w196 -> [w217]
              n48 = Divide(x=w220, y=w219) -> (x/y=w218:dbl)
              n49 = for {
                N: w219 -> [_]
                shift-right: [w225] -> w221
                shift-left: w222 -> [w226]
                tunnel: w218 -> [w224]
                tunnel: w217 -> [w223]
                n50 = formula code="h=h*0.5;\n//cromer 1\nx[0]=x[0]+h*(-b[0]*x[0]-4*(x[1]+x[2])-x[1]*x[1]);\nx[1]=x[1]+h*(-b[1]*x[1]-4*(x[0]+x[2])-x[2]*x[2]);\nx[2]=x[2]+h*(-b[2]*x[2]-4*(x[1]+x[0])-x[0]*x[0]);\n//D2\nx[2]=(x[2]+h*(-4*(x[1]+x[0])-x[0]*x[0]))/(1+b[0]*h);\nx[1]=(x[1]+h*(-4*(x[0]+x[2])-x[2]*x[2]))/(1+b[1]*h);\nx[0]=(x[0]+h*(-4*(x[1]+x[2])-x[1]*x[1]))/(1+b[2]*h);"("x"=w226, "h"=w224, "b"=w223) -> ("x"=w225:dbl[])
              }
            }
            n51 = call "Extrapolator_Lorenz.vi"("Порядок экстраполятора"=2 ("input variable"), "Dimension"=3 ("input variable"), "Ext.Type"=w215, "Х - нач. условия"=w211, "n"=w216, "k"=w209) -> ("TPrev"=w193:dbl[], "Tout"=w194:dbl[])  [unwired: 4 in]
            n52 = Subtract(x=w194, y=w193) -> (x-y=w195:dbl[])
            n53 = Equal?(x=w200, y=10) -> (x = y?=w202:bool)
            n54 = call-poly <vilib>:"Vector Norm.vi"("Input Vector"=w195) -> ("norm"=w192:dbl)  [unwired: 9 in, 1 out]
            n55 = call "Common_StepVariator.vi"("err"=w192, "tolerance"=w206, "Hmax"=w207, "Шаг h, с"=w197, "Current time"=w205, "k"=w209, "Hmin"=w208, "tmax"=w204) -> ("Hnew"=w210:dbl, "New time"=w198:dbl, "stop"=w199:bool)  [unwired: 4 in, 1 out]
            n56 = Or(x=w202, y=w199) -> (x .or. y?=w201:bool)
          }
        }
      }
      frame #2 {
        n57 = call <vilib>:"High Resolution Relative Seconds.vi"() -> ("relative seconds"=w227:dbl)
      }
    }
    n58 = Subtract(x=w145, y=w144) -> (x-y=w143:dbl)
  }
  "Step time variation" <- w20
  n59 = case shown="True" TRUE {
    tunnel: w20 -> [w228 w231]
    tunnel: [w229 w230] -> w19
    frame False {
      n60 = call-poly <vilib>:"RMS.vi"("X"=w228) -> ("rms value"=w229:dbl)  [unwired: 1 out]
    }
    frame True {
      n61 = call <vilib>:"Median.vi"("X"=w231) -> ("median"=w230:dbl)  [unwired: 1 out]
    }
  }
  "Elapsed Time" <- w19
